vi "Init_QuWire.vi"(8 "error in (no error)":errorcluster, 11 "QuWire in":refnum<class "QuWire.lvclass">) -> (0 "error out":errorcluster, 3 "QuWire out":refnum<class "QuWire.lvclass">)   [LabVIEW 2020, in "QuWire.lvclass"]
uses:
  QuWire.lvclass
  QuWire.lvclass/QuWire.ctl
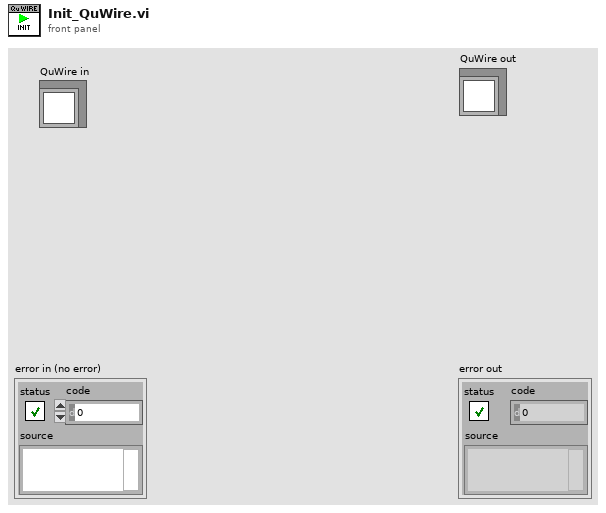
[diagram p1: front panel]
types:
  T1 = cluster{"queue out":refnum<queue>, "notifier out":refnum<notifier>}
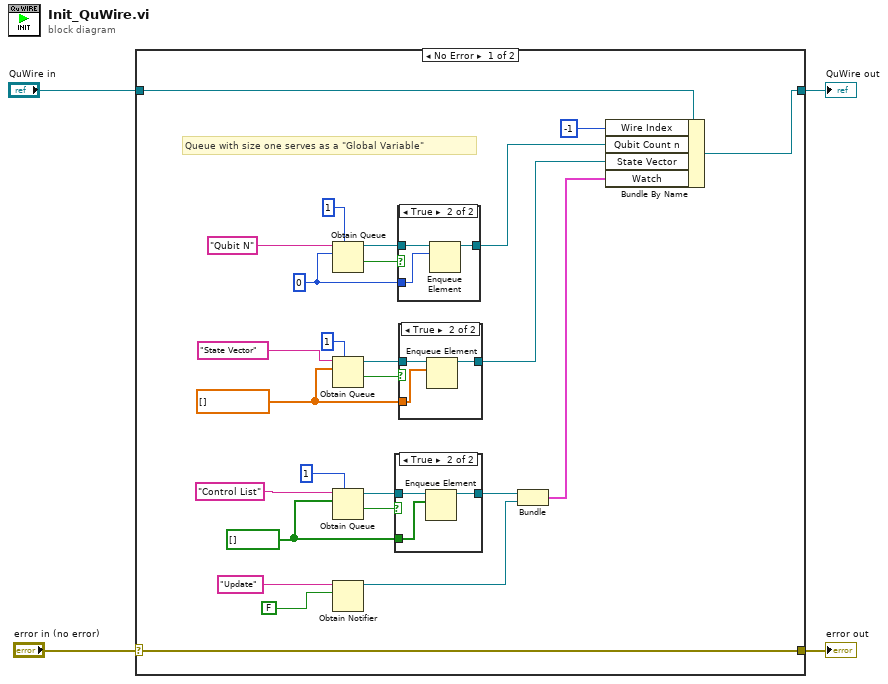
[diagram p0: block diagram]
diagram:
  n1 = case shown="No Error" "error in (no error)" {
    selector: "error in (no error)" -> [w30 w44]
    tunnel: [w30 w44] -> w3
    tunnel: [w28 w43] -> w1
    tunnel: "QuWire in" -> [w29 w43]
    frame No Error {
      w13 = bool[] [] ("Boolean")
      w20 = cdb[] [] ("subarray")
      w19 = 0 ("# Qubits")
      # "Queue with size one serves as a \"Global Variable\""
      n2 = Obtain Queue(max queue size (-1, unlimited)=1, name (unnamed)="Qubit N", element data type=w19) -> (queue out=w15:refnum<queue>, created new?=w7:bool)  [unwired: 2 in, 1 out]
      n3 = Obtain Queue(max queue size (-1, unlimited)=1, name (unnamed)="State Vector", element data type=w20) -> (queue out=w22:refnum<queue>, created new?=w6:bool)  [unwired: 2 in, 1 out]
      n4 = Obtain Queue(max queue size (-1, unlimited)=1, name (unnamed)="Control List", element data type=w13) -> (queue out=w16:refnum<queue>, created new?=w5:bool)  [unwired: 2 in, 1 out]
      n5 = Obtain Notifier(name (unnamed)="Update", notification data type=FALSE) -> (notifier out=w9:refnum<notifier>)  [unwired: 2 in, 2 out]
      n6 = case shown="True" w5 {
        tunnel: w16 -> [w31 w34]
        tunnel: w13 -> [_ w33]
        tunnel: [w31 w32] -> w10
        frame False {
        }
        frame True {
          n7 = Enqueue Element(queue=w34, element=w33) -> (queue out=w32:refnum<queue>)  [unwired: 2 in, 2 out]
        }
      }
      n8 = case shown="True" w7 {
        tunnel: w19 -> [_ w42]
        tunnel: w15 -> [w39 w41]
        tunnel: [w39 w40] -> w14
        frame False {
        }
        frame True {
          n9 = Enqueue Element(queue=w41, element=w42) -> (queue out=w40:refnum<queue>)  [unwired: 2 in, 2 out]
        }
      }
      n10 = case shown="True" w6 {
        tunnel: w22 -> [w35 w38]
        tunnel: [w35 w37] -> w21
        tunnel: w20 -> [_ w36]
        frame False {
        }
        frame True {
          n11 = Enqueue Element(queue=w38, element=w36) -> (queue out=w37:refnum<queue>)  [unwired: 2 in, 2 out]
        }
      }
      n12 = Bundle("queue out"=w10, "notifier out"=w9) -> (w8:T1)  [unwired: 1 in]
      n13 = Bundle By Name(cluster=w29, "Wire Index"=-1, "Qubit Count n"=w14, "State Vector"=w21, "Watch"=w8) -> (w28:refnum<class "QuWire.lvclass">)
    }
    frame Error {
    }
  }
  "error out" <- w3
  "QuWire out" <- w1
